vi "GetTemperature.vi"(10 "HeaterIn":dbl, 11 "PyroIn":dbl) -> (2 "HeaterTemp":dbl, 3 "PyroTemp":dbl)   [LabVIEW 2020]
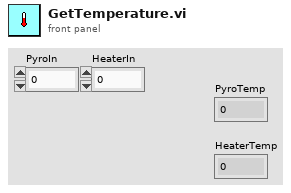
[diagram p1: front panel]
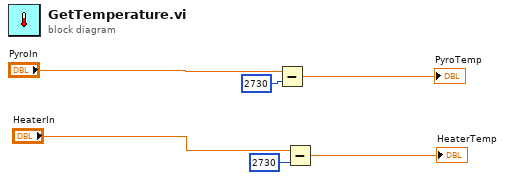
[diagram p0: block diagram]
diagram:
  n1 = Subtract(x="PyroIn", y=u16 2730 ("Starting Address")) -> (x-y=→"PyroTemp":dbl)
  n2 = Subtract(x="HeaterIn", y=u16 2730 ("Starting Address")) -> (x-y=→"HeaterTemp":dbl)
